vi "Calculate Extinction.vi"(8 "error in":errorcluster, 11 "CRDS Cell in":refnum<class "CRDS Cell.lvclass">) -> (0 "error out":errorcluster, 3 "CRDS Cell out":refnum<class "CRDS Cell.lvclass">)   [LabVIEW 2015, in "CRDS Cell.lvclass"]
uses:
  CRDS Cell.lvclass
  CRDS Cell.lvclass/CRDS Cell.ctl
  Data/Cell/CRDS Cell Data.lvclass/CRDS Cell Data.ctl
  Data/Cell/Read extParam.vi
  Data/Cell/Write extParam.vi
  Data/Cell/Read hkParam.vi
  Data/Cell/CRDS Cell Data.lvclass
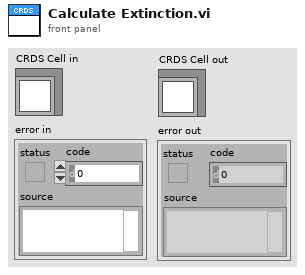
[diagram p1: front panel]
types:
  T1 = typedef "extparam.ctl" = cluster{"Tau":sgl, "Tau0cor":sgl, "ext":sgl, "extCorr":sgl, "stdevTau":sgl, "eTau":sgl, "taucorr":sgl, "Tau0":sgl, "max":sgl}
  T2 = typedef "calData.ctl" = cluster{"rhDilFac":sgl, "Q":sgl, "Tmean":sgl, "extDilFac":sgl, "rhCell":sgl, "P":sgl, "T":sgl}
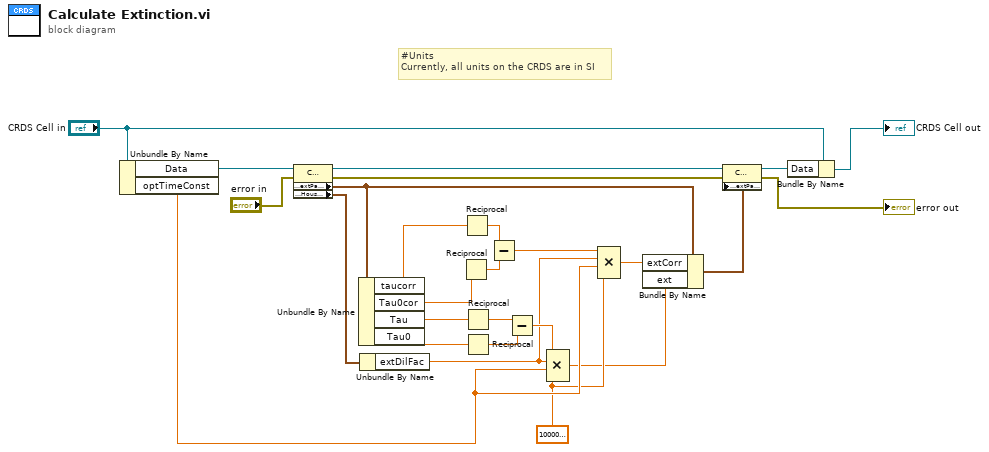
[diagram p0: block diagram]
diagram:
  w12 = sgl 1000000.0 ("value")
  # "#Units\nCurrently, all units on the CRDS are in SI"
  n1 = Unbundle By Name("CRDS Cell in") -> ("Data"=w26:refnum<class "CRDS Cell Data.lvclass">, "optTimeConst"=w13:sgl)
  n2 = property class="CRDS Cell"(reference=w26, error in="error in") -> (reference out=w8:refnum<class "CRDS Cell Data.lvclass">, error out=w7:errorcluster, "Data Access:extParam"=w10:T1, "Data Access:Housekeeping"=w21:T2)
  n3 = Unbundle By Name(w10) -> ("taucorr"=w17:sgl, "Tau0cor"=w16:sgl, "Tau"=w25:sgl, "Tau0"=w24:sgl)
  n4 = Unbundle By Name(w21) -> ("extDilFac"=w14:sgl)
  n5 = Reciprocal(x=w16) -> (1/x=w19:sgl)
  n6 = Reciprocal(x=w17) -> (1/x=w18:sgl)
  n7 = Reciprocal(x=w25) -> (1/x=w23:sgl)
  n8 = Reciprocal(x=w24) -> (1/x=w22:sgl)
  n9 = Subtract(x=w18, y=w19) -> (x-y=w15:sgl)
  n10 = Subtract(x=w23, y=w22) -> (x-y=w20:sgl)
  n11 = Compound Arithmetic op=MULTIPLY(w20, w14, w13, w12) -> (w4:sgl)
  n12 = Compound Arithmetic op=MULTIPLY(w15, w14, w13, w12) -> (w5:sgl)
  n13 = Bundle By Name(cluster=w10, "extCorr"=w5, "ext"=w4) -> (w9:T1)
  n14 = property class="CRDS Cell"(reference=w8, error in=w7, "Data Access:extParam"=w9) -> (reference out=w3:refnum<class "CRDS Cell Data.lvclass">, error out=→"error out":errorcluster)
  n15 = Bundle By Name(cluster="CRDS Cell in", "Data"=w3) -> (→"CRDS Cell out":refnum<class "CRDS Cell.lvclass">)
